vi "Message Globals.vi"() -> ()   [LabVIEW 2019]
panel:
  out "Sensor Connected?":bool
  in  "Last Heart Beat Time":timestamp
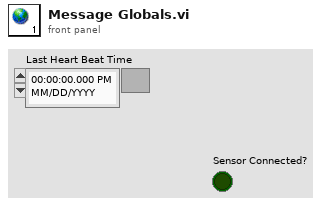
[diagram p1: front panel]
diagram:
